vi "Start.vi"(8 "error in (no error)":errorcluster, 11 "NI SMU in":refnum<class "NI SMU.lvclass">) -> (0 "error out":errorcluster, 3 "NI SMU out":refnum<class "NI SMU.lvclass">)   [LabVIEW 2020, in "NI SMU.lvlib" / "NI SMU.lvclass"]
uses:
  NI SMU.lvclass
  NI SMU.lvclass/NI SMU.ctl
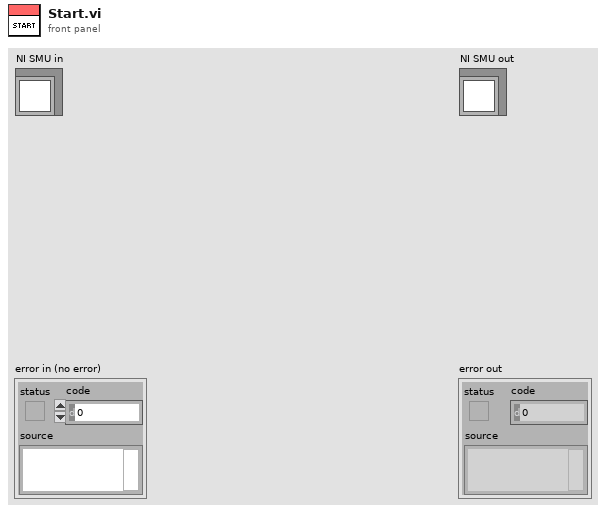
[diagram p1: front panel]
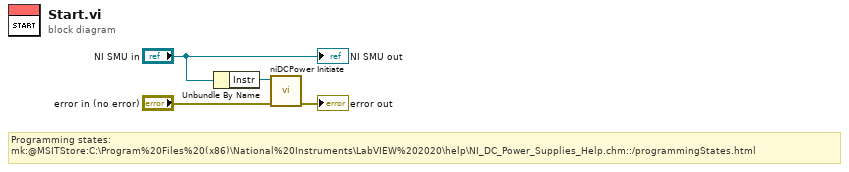
[diagram p0: block diagram]
diagram:
  # "Programming states:\nmk:@MSITStore:C:\\Program%20Files%20(x86)\\National%20Instruments\\LabVIEW%202020\\help\\NI_DC_Power_Supplies_Help.chm::/programmingStates.html"
  n1 = Unbundle By Name("NI SMU in") -> ("Instr"=w4:refnum<k15>)
  n2 = call <instrlib>:"niDCPower Initiate.vi"("error in (no error)"="error in (no error)", "instrument handle"=w4) -> ("error out"=→"error out":errorcluster)  [unwired: 8 in, 1 out]
  "NI SMU out" <- "NI SMU in"
